vi "PC Rio Data passing test.vi"() -> ()   [LabVIEW 2017]
panel:
  in  "PC To Rio":T1
  # "Max X 400mm"
  # "Max Y 600mm"
  # "Max Enery 10mJ"
  # "90 is facing goal\n0 anti clockwise\n180 clockwise"
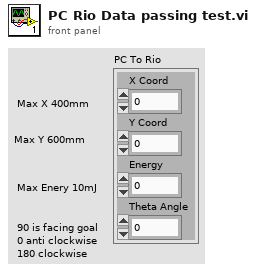
[diagram p1: front panel]
types:
  T1 = cluster{"X Coord":dbl, "Y Coord":dbl, "Energy":dbl, "Theta Angle":dbl}
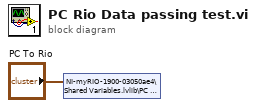
[diagram p0: block diagram]
diagram:
  n1 = shared-variable "NI-myRIO-1900-03050ae4\\Shared Variables.lvlib\\PC To Rio"("PC To Rio") -> ()  [unwired: 1 in, 1 out]
